vi "시간 저장(SubVI).vi"   [LabVIEW 2014]
uses:
  <vilib>/Utility/sysdir.llb/System Directory Type.ctl
types:
  T1 = enum16{"open", "replace", "create", "open or create", "replace or create", "replace or create with confirmation"}
  T2 = typedef "System Directory Type.ctl" = i32
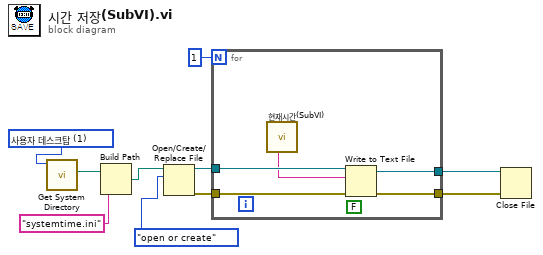
[diagram p0: block diagram]
diagram:
  w8 = T2 1 items=["사용자 홈"=0, "사용자 데스크탑"=1, "사용자 문서"=2, "사용자 어플리케이션 데이터"=3, "사용자 환경"=4, "사용자 임시"=5, "퍼블릭 문서"=6, "퍼블릭 어플리케이션 데이터"=7, "퍼블릭 환경"=8, "퍼블릭 캐시"=13, "시스템 코어 라이브러리"=9, "시스템 설치된 라이브러리"=10, "어플리케이션 파일"=11, "부팅 볼륨 루트"=12] ("system directory type")
  n1 = call <vilib>:"Get System Directory.vi"("system directory type"=w8) -> ("system directory"=w3:path)  [unwired: 10 in]
  n2 = Build Path(base path=w3, name or relative path="systemtime.ini" ("이름 또는 상대 경로")) -> (appended path=w5:path)
  n3 = Open/Create/Replace File(file path (use dialog)=w5, operation (0:open)=T1."open or create" ("동작(0:open)")) -> (refnum out=w7:refnum<file>, error out=w6:errorcluster)  [unwired: 4 in, 1 out]
  n4 = for {
    N: 1 -> [_]
    tunnel: w6 -> [w15]
    tunnel: [w14] -> w1
    tunnel: [w13] -> w2
    tunnel: w7 -> [w12]
    (unwired) FALSE
    n5 = call "현재시간(SubVI).vi"() -> ("시 문자열"=w11:string)  [unwired: 5 in, 6 out]
    n6 = Write to Text File(file (use dialog)=w12, text=w11, error in=w15) -> (refnum out=w13:refnum<file>, error out=w14:errorcluster)  [unwired: 1 in, 1 out]
  }
  n7 = Close File(refnum=w2, error in=w1) -> ()  [unwired: 2 out]
